vi "Parse resolv.conf.vi"(8 "error in (no error)":errorcluster, 11 "resolv.conf contents":string) -> (0 "error out":errorcluster, 3 "DNS server addresses":refnum<class "Generic Network Address.lvclass">[](array[class]))   [LabVIEW 2020, in "NI_WFCN.lvlib" / "Hostname Network Address.lvclass"]
doc: "Parse resolv.conf contents and return the first configured DNS server address, if it exists."
uses:
  <vilib>/net/WFCN/Addressing/Hostname Network Address/Hostname Network Address.lvclass
  <vilib>/net/WFCN/Addressing/Generic Network Address/Generic Network Address.lvclass
  <vilib>/net/WFCN/Addressing/IPv4 Network Address/IPv4 Network Address.lvclass/IPv4 Network Address.ctl
  <vilib>/net/WFCN/Addressing/Generic Network Address/Generic Network Address.lvclass/Generic Network Address.ctl
  <vilib>/net/WFCN/Addressing/Hostname Network Address/Hostname Network Address.lvclass/Hostname Network Address.ctl
  <vilib>/net/WFCN/Addressing/Hostname Network Address/Create from string.vi
  <vilib>/net/WFCN/Utility/Is IPv4 address.vi
  <vilib>/net/WFCN/Addressing/IPv4 Network Address/Create from U32.vi
  <vilib>/net/WFCN/Addressing/Generic Network Address/Create for unparsable.vi
  <vilib>/net/WFCN/Utility/Is hostname mDNS.vi
  <vilib>/dlg_ctls.llb/Space Constant.vi
  <vilib>/net/WFCN/Addressing/IPv4 Network Address/IPv4 Network Address.lvclass
  e:/builds/penguin/labview/branches/2020/dev/dist/vi.lib/net/WFCN/Addressing/Generic Network Address/Generic Network Address.lvclass
  <vilib>/net/WFCN/Addressing/mDNS Hostname Network Address/mDNS Hostname Network Address.lvclass
  e:/builds/penguin/labview/branches/2020/dev/dist/vi.lib/net/WFCN/Addressing/Hostname Network Address/Hostname Network Address.lvclass
  <vilib>/Utility/error.llb/Error Cluster From Error Code.vi
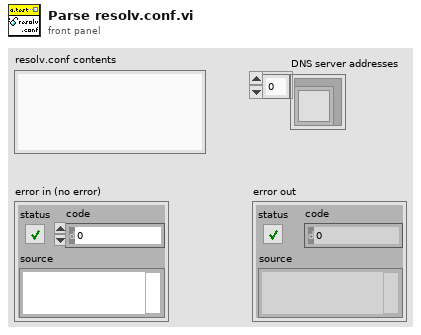
[diagram p1: front panel]
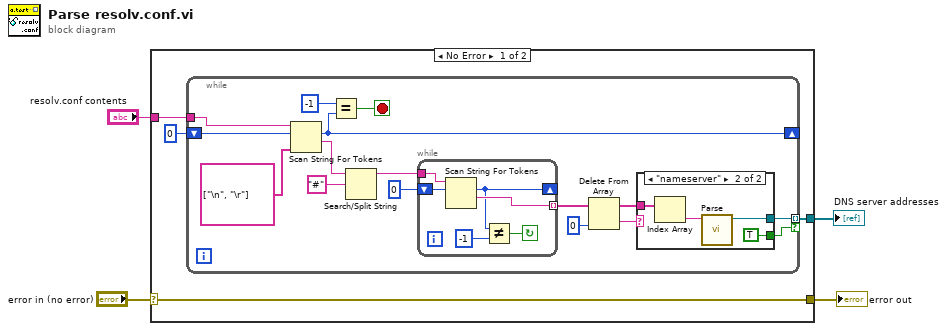
[diagram p0: block diagram]
diagram:
  n1 = case shown="No Error" "error in (no error)" {
    selector: "error in (no error)" -> [w5 w35]
    tunnel: "resolv.conf contents" -> [w8 _]
    tunnel: [w6 _] -> w3
    tunnel: [w5 w35] -> w1
    frame No Error {
      n2 = while {
        tunnel: w8 -> [w12]
        shift-right: [w9] -> _
        shift-left: 0 -> [w11]
        tunnel: [w17] -> w6 mode=indexing if=w14
        stop <- w16 stop-if-true
        n3 = Scan String For Tokens(6:string[] ["\n", "\r"], 8:w11, 9:w12) -> (1:w10:string, 2:w9:i32)  [unwired: 3 in, 2 out]
        n4 = Equal?(x=-1 ("y"), y=w9) -> (x = y?=w16:bool)
        n5 = Search/Split String(string=w10, search string/char (-)="#") -> (substring before match=w23:string)  [unwired: 1 in, 2 out]
        n6 = while {
          tunnel: w23 -> [w34]
          shift-right: [w31] -> _
          shift-left: 0 ("offset past token") -> [w33]
          tunnel: [w32] -> w21 mode=indexing
          stop <- w29 continue-if-true
          n7 = Scan String For Tokens(8:w33, 9:w34) -> (1:w32:string, 2:w31:i32)  [unwired: 4 in, 2 out]
          n8 = Not Equal?(x=w31, y=-1) -> (x != y?=w29:bool)
        }
        n9 = Delete From Array(array=w21, index=0) -> (deleted portion=w19:string, array with subset deleted=w18:string[])  [unwired: 1 in]
        n10 = case shown="\"nameserver\"" w19 {
          tunnel: w18 -> [_ w28]
          tunnel: [_ w26] -> w17
          tunnel: [_ TRUE] -> w14
          frame Default {
          }
          frame "nameserver" {
            n11 = Index Array(array=w28) -> (element=w27:string)  [unwired: 1 in]
            n12 = call <vilib>:"Parse.vi"("address string"=w27) -> ("address"=w26:refnum<class "Generic Network Address.lvclass">)  [unwired: 10 in]
          }
        }
      }
    }
    frame Error {
    }
  }
  "error out" <- w1
  "DNS server addresses" <- w3
